vi "GenerateCode.vi"(1 "Terms":T1[](array[typedef]), 3 "Diagram":refnum<vi>, 5 "XRef":refnum<vi>, 6 "State In":T4={"Input Type"=variant(dbl 0.0), "Width"=0, "Typedef Name"="", "Value Type"=variant, "Selection"=0, "Options"=[], "Selections"=[], "Display Selections"=[], "Element Names"=[], "Typedef Name Width"=0, "Display Selection Width"=[], "Code Generated"=FALSE, "Is DVR"=FALSE, "Write Lock"=FALSE}) -> (0 "Generated Code?":bool, 2 "State Out":T4={"Input Type"=variant(dbl 0.0), "Width"=0, "Typedef Name"="", "Value Type"=variant, "Selection"=0, "Options"=[], "Selections"=[], "Display Selections"=[], "Element Names"=[], "Typedef Name Width"=0, "Display Selection Width"=[], "Code Generated"=FALSE, "Is DVR"=FALSE, "Write Lock"=FALSE}, 4 "Reply":string[](array[string]))   [LabVIEW 2015, in "Read-Write-Signals.xnode"]
doc: "This ability VI is called when it is time to define the execution behavior of your XNode via LabVIEW's scripting API. This VI is only called when you have previously informed LabVIEW that you need to script through a GenerateCode reply. Diagram is a reference to a diagram of a temporary VI. This diagram contains exactly one front panel terminal for each terminal of your XNode. Terms is an array of pairs of Term IDs and terminal references. LabVIEW will copy code scripted into this diagram into your XNode and connect everything to the correct terminals. The front panel terminals that are on this diagram are special in that they can only be on the top level diagram.\n \n Generate Code? is used to tell LabVIEW whether or not you want to copy the scripted diagram over. If there is an error and you wish not to commit the changes, then the old XNode behavior will be left unchanged. If you set Generate Code? to false, then this VI will be called again next time type propagation is run. Otherwise, it will not be called until you indicate that it should be through the reply on another ability VI.\n \n Because the diagram you are scripting into is separate from the VI containing the XNode instance, type propagation and the data manager will run on the temporary VI after each scripting call.\n \n You should not use the Copy scripting method to move code into the temporary VI. This will adversely affect the user's clipboard. You should use the Move scripting method instead.\n\nDefault behavior: None.\n\nThis ability does not provide UI and OS messages are not handled.\n\nSee also: ModifyCode"
uses:
  Read-Write-Signals.xnode
  State.ctl
  Read-Write-Signals Item.ctl
  Read-Write-Signals Sub Item.ctl
  Read-Write-Signals Sub Item Type.ctl
  Read-Write-Signals Selection.ctl
  Read-Write-Signals Display Selection.ctl
  <vilib>/XNodeSupport/XNodeTermIDPair.ctl
  <vilib>/XNodeSupport/XNodeTermRef.ctl
  <vilib>/XNodeSupport/XNodeString.ctl
  <vilib>/Erdos Miller/LV-Scripting/LV-Scripting.lvlib
  <vilib>/Utility/Data Type/NI_Data Type.lvlib
  <vilib>/XNodeSupport/NI_XNodeSupport.lvlib
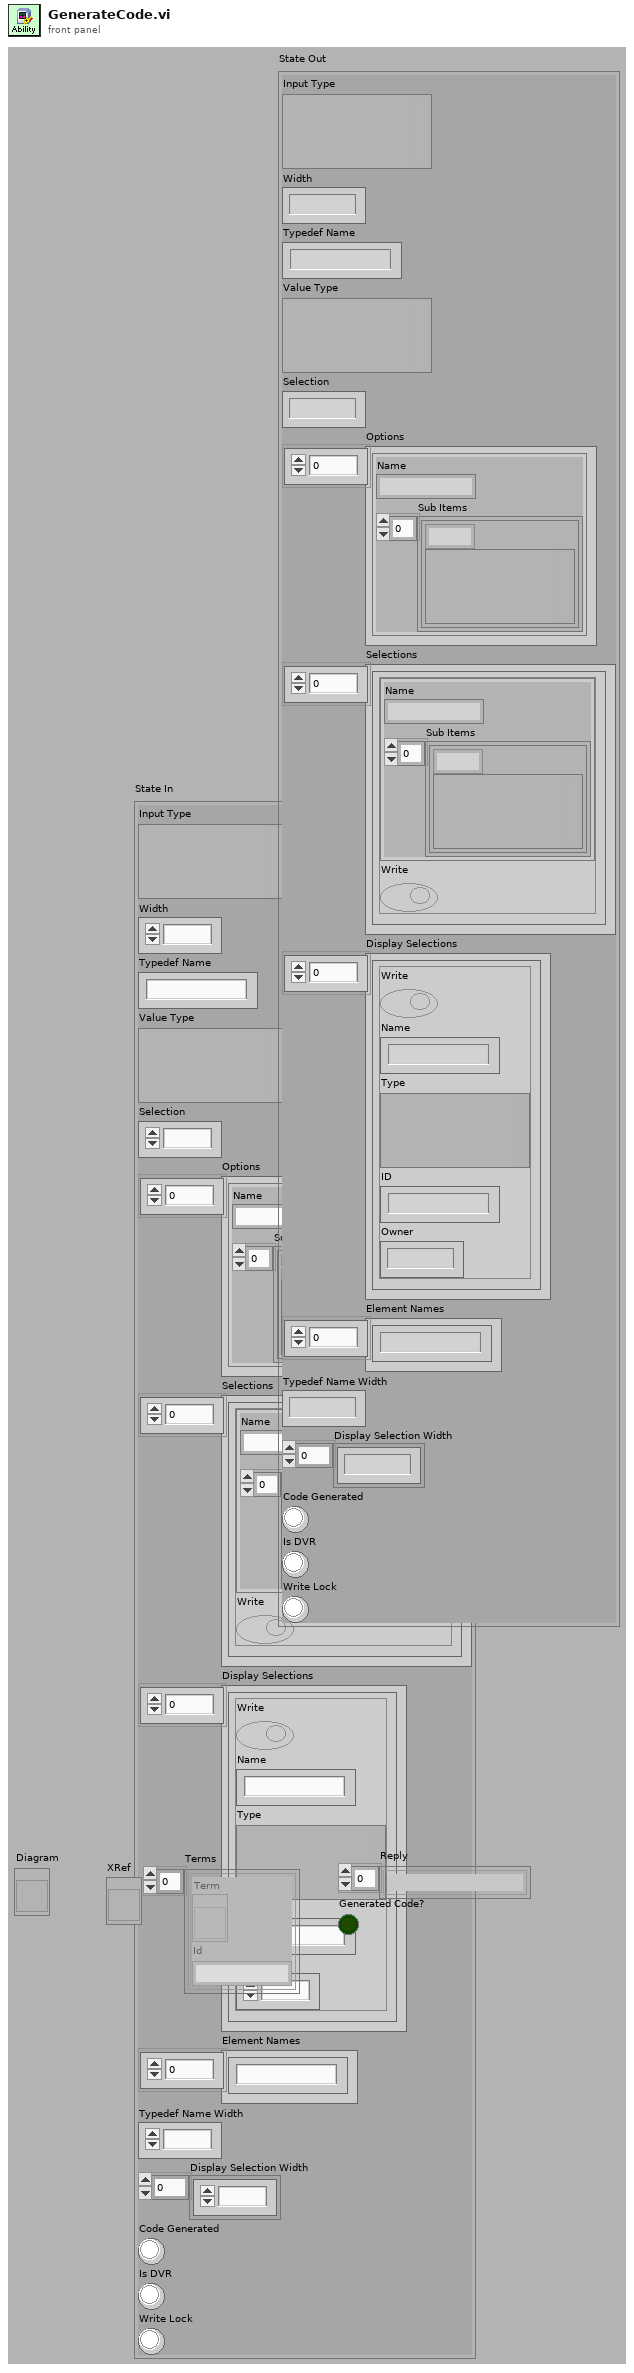
[diagram p1: front panel]
types:
  T1 = typedef "NI_XNodeSupport.lvlib/XNodeTermIDPair.ctl" = cluster{"Term":T2, "Id":T3}
  T2 = typedef "NI_XNodeSupport.lvlib/XNodeTermRef.ctl" = refnum<vi>
  T3 = typedef "NI_XNodeSupport.lvlib/XNodeString.ctl" = string
  T4 = typedef "Read-Write-Signals.xnode/State.ctl" = cluster{"Input Type":variant, "Width":i32, "Typedef Name":string, "Value Type":variant, "Selection":i32, "Options":T5[], "Selections":T8[], "Display Selections":T9[], "Element Names":string[], "Typedef Name Width":i32, "Display Selection Width":i32[], "Code Generated":bool, "Is DVR":bool, "Write Lock":bool}
  T5 = typedef "Read-Write-Signals Item.ctl" = cluster{"Name":string, "Sub Items":T6[]}
  T6 = typedef "Read-Write-Signals Sub Item.ctl" = cluster{"Type":T7, "Value":variant}
  T7 = typedef "Read-Write-Signals Sub Item Type.ctl" = enum8{"Cluster Element", "Array Element", "Subarray"}
  T8 = typedef "Read-Write-Signals Selection.ctl" = cluster{"Item":T5, "Write":bool}
  T9 = typedef "Read-Write-Signals Display Selection.ctl" = cluster{"Write":bool, "Name":string, "Type":variant, "ID":string, "Owner":i32}
  T10 = typedef "NI_Data Type.lvlib/Data Type.ctl" = enum8{"Invalid Type", "Void", "I8", "I16", "I32", "I64", "U8", "U16", "U32", "U64", "Single Float", "Double Float", "Extended Float", "Single Complex", "Double Complex", "Extended Complex", "Enum U8", "Enum U16", "Enum U32", "Enum U64", "Single Float With Unit", "Double Float With Unit", "Extended Float With Unit", "Single Complex with Unit", "Double Complex with Unit", "Extended Complex with Unit", "Boolean", "String", "Path", "Picture", "Tag", "Array", "Cluster", "Variant", "LV Variant", "Waveform", "Timestamp", "Digital Waveform", "Digital Data", "ExpressData", "Refnum", "External Data", "VI", "Poly VI", "LabVIEW Class Instance", "Fixed Point"}
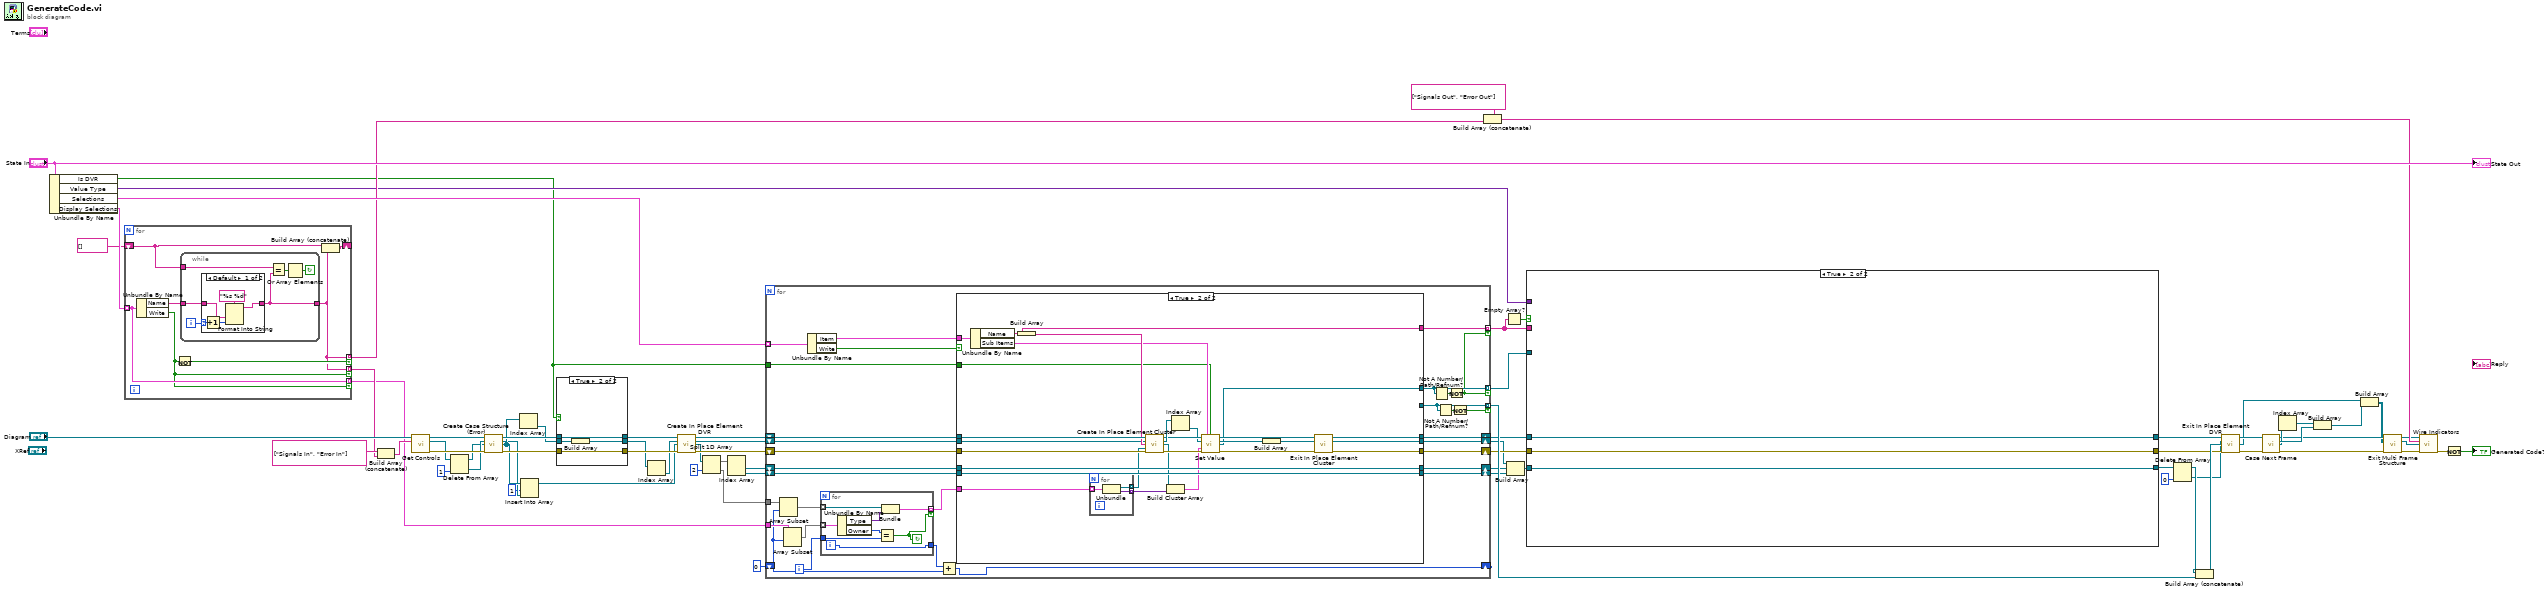
[diagram p0: block diagram]
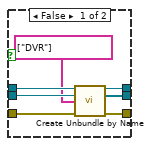
[diagram p2: hidden frame]
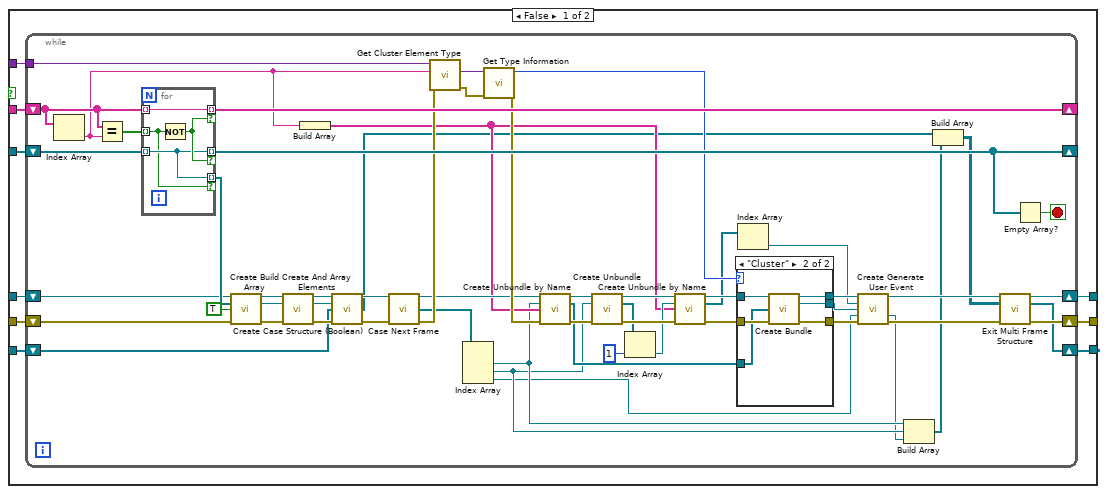
[diagram p3: hidden frame]
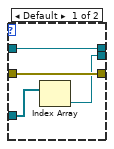
[diagram p4: hidden frame]
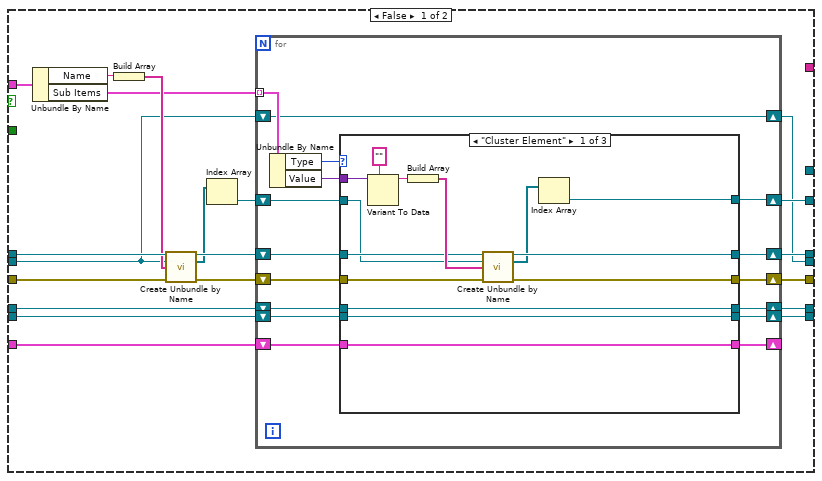
[diagram p5: hidden frame]
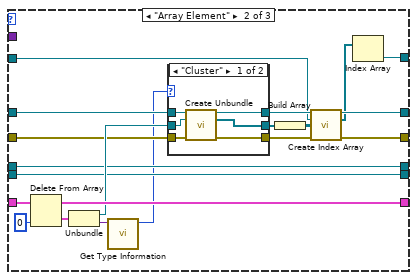
[diagram p6: hidden frame]
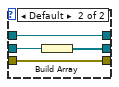
[diagram p7: hidden frame]
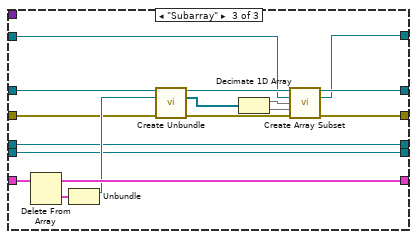
[diagram p8: hidden frame]
diagram:
  n1 = Unbundle By Name("State In") -> ("Is DVR"=w25:bool, "Value Type"=w41:variant, "Selections"=w63:T8[], "Display Selections"=w54:T9[])
  n2 = for {
    tunnel: w54 -> [w75] mode=indexing
    tunnel: [w76] -> w50 mode=indexing if=w80
    tunnel: [w76] -> w70 mode=indexing if=w74
    tunnel: [w75] -> w27 mode=indexing if=w74
    shift-right: [w79] -> _
    shift-left: string[] [] -> [w78]
    n3 = Unbundle By Name(w75) -> ("Name"=w77:string, "Write"=w74:bool)
    n4 = Not(x=w74) -> (.not. x?=w80:bool)
    n5 = while {
      tunnel: w77 -> [w84]
      tunnel: w78 -> [w86]
      tunnel: [w81] -> w76
      i -> [w85]
      stop <- w82 continue-if-true
      n6 = case shown="Default" w85 {
        selector: w85 -> [w90 _]
        tunnel: w84 -> [w89 w92]
        tunnel: [w88 w92] -> w81
        frame Default {
          n7 = Increment(x=w90) -> (x+1=w87:i32)
          n8 = Format Into String(format string="%s %d", w89, w87) -> (resulting string=w88:string)  [unwired: 2 in, 1 out]
        }
        frame 0 {
        }
      }
      n9 = Equal?(x=w86, y=w81) -> (x = y?=w83:bool[])
      n10 = Or Array Elements(Boolean array=w83) -> (logical OR=w82:bool)
    }
    n11 = Build Array (concatenate)(w78, w76) -> (w79:string[])
  }
  n12 = Build Array (concatenate)(string[] ["Signals In", "Error In"] ("Control Names"), w70) -> (w69:string[])
  n13 = call <vilib>:"Get Controls.vi"("Diagram in"="Diagram", "Control Names"=w69) -> ("Diagram out"=w23:refnum<vi>, "Control Terminals"=w18:refnum<vi>[], "error out"=w68:errorcluster)  [unwired: 11 in]
  n14 = Delete From Array(array=w18, index=1) -> (deleted portion=w21:refnum<vi>, array with subset deleted=w20:refnum<vi>[])  [unwired: 1 in]
  n15 = call <vilib>:"Create Case Structure (Error).vi"("Diagram in"=w23, "Selector"=w21, "Inputs"=w20, "error in (no error)"=w68) -> ("Selected Diagram"=w22:refnum<vi>, "Selector"=w3:refnum<vi>, "Inputs"=w4:refnum<vi>[], "error out"=w24:errorcluster)  [unwired: 8 in]
  n16 = Index Array(array=w4) -> (element=w19:refnum<vi>)  [unwired: 1 in]
  n17 = Insert Into Array(array=w4, index=1, new element=w3) -> (w1:refnum<vi>[])
  n18 = case shown="True" w25 {
    tunnel: w22 -> [w99 w103]
    tunnel: w24 -> [w98 w102]
    tunnel: w19 -> [w97 w101]
    tunnel: [w95 w103] -> w67
    tunnel: [w94 w102] -> w66
    tunnel: [w93 w100] -> w65
    frame False {
      n19 = call <vilib>:"Create Unbundle by Name.vi"("Diagram in"=w99, "input cluster"=w97, "Element Names"=string[] ["DVR"], "error in (no error)"=w98) -> ("Diagram out"=w95:refnum<vi>, "Outputs"=w93:refnum<vi>[], "error out"=w94:errorcluster)  [unwired: 9 in]
    }
    frame True {
      n20 = Build Array(w101) -> (w100:refnum<vi>[])
    }
  }
  n21 = Index Array(array=w65) -> (element=w64:refnum<vi>)  [unwired: 1 in]
  n22 = call <vilib>:"Create In Place Element DVR.vi"("Diagram in"=w67, "DVR"=w64, "Inputs"=w1, "error in (no error)"=w66) -> ("Diagram out"=w62:refnum<vi>, "Data Value"=w60:refnum<vi>, "Inputs"=w56:refnum<vi>[], "error out"=w61:errorcluster)  [unwired: 7 in, 1 out]
  n23 = Split 1D Array(array=w56, index=2) -> (first subarray=w55:refnum<vi>[], second subarray=w28:refnum<vi>[])
  n24 = Index Array(array=w55) -> (element #1=w58:refnum<vi>, element #2=w59:refnum<vi>)  [unwired: 2 in]
  n25 = for {
    tunnel: w63 -> [w131] mode=indexing
    shift-right: [w125] -> w42
    shift-left: w62 -> [w130]
    shift-right: [w124] -> w43
    shift-left: w61 -> [w129]
    shift-right: [w122] -> w39
    shift-left: w59 -> [w126]
    shift-right: [w123] -> w40
    shift-left: w58 -> [w127]
    tunnel: [w119] -> w53 mode=indexing if=w120
    shift-right: [w118] -> w38
    shift-left: w60 -> [w128]
    tunnel: [w116] -> w44 mode=indexing if=w114
    tunnel: [w115] -> w46 mode=indexing if=w114
    tunnel: w28 -> [w109]
    tunnel: w27 -> [w111]
    shift-right: [w107] -> _
    shift-left: 0 -> [w105]
    tunnel: w25 -> [w104]
    i -> [w113]
    n26 = Array Subset(array=w109, index=w105) -> (w108:refnum<vi>[])  [unwired: 1 in]
    n27 = Array Subset(array=w111, index=w105) -> (w110:T9[])  [unwired: 1 in]
    n28 = Unbundle By Name(w131) -> ("Item"=w132:T5, "Write"=w133:bool)
    n29 = for {
      tunnel: w108 -> [w137] mode=indexing
      tunnel: w110 -> [w141] mode=indexing
      tunnel: w113 -> [w139]
      tunnel: [w136] -> w112 mode=indexing if=w135
      tunnel: [w134] -> w106
      i -> [w134]
      stop <- w135 continue-if-true
      n30 = Unbundle By Name(w141) -> ("Type"=w138:variant, "Owner"=w140:i32)
      n31 = Equal?(x=w140, y=w139) -> (x = y?=w135:bool)
      n32 = Bundle(w137, "Type"=w138) -> (w136:cluster{refnum<vi>, "Type":variant})  [unwired: 1 in]
    }
    n33 = Add(x=w106, y=w105) -> (x+y=w107:i32)
    n34 = case shown="True" w133 {
      tunnel: w132 -> [w161 w265]
      tunnel: w130 -> [w160 w263]
      tunnel: w129 -> [w157 w261]
      tunnel: w128 -> [w143 w258]
      tunnel: w112 -> [w151 w245]
      tunnel: w127 -> [w150 w247]
      tunnel: w126 -> [w149 w248]
      tunnel: [w148 w256] -> w125
      tunnel: [w147 w257] -> w124
      tunnel: [w146 w247] -> w123
      tunnel: [w145 w248] -> w122
      tunnel: [w144 _] -> w119
      tunnel: [w142 w255] -> w118
      tunnel: [_ w241] -> w116
      tunnel: [_ w240] -> w115
      tunnel: w104 -> [_ w239]
      frame False {
        n35 = Unbundle By Name(w161) -> ("Name"=w159:string, "Sub Items"=w156:T6[])
        n36 = Build Array(w159) -> (w158:string[])
        n37 = call <vilib>:"Create Unbundle by Name.vi"("Diagram in"=w160, "input cluster"=w143, "Element Names"=w158, "error in (no error)"=w157) -> ("Diagram out"=w155:refnum<vi>, "Outputs"=w153:refnum<vi>[], "error out"=w154:errorcluster)  [unwired: 9 in]
        n38 = Index Array(array=w153) -> (element=w152:refnum<vi>)  [unwired: 1 in]
        n39 = for {
          tunnel: w156 -> [w177] mode=indexing
          shift-right: [w167] -> _
          shift-left: w151 -> [w174]
          shift-right: [w166] -> w148
          shift-left: w155 -> [w173]
          shift-right: [w165] -> w147
          shift-left: w154 -> [w172]
          shift-right: [w169] -> w146
          shift-left: w150 -> [w170]
          shift-right: [w168] -> w145
          shift-left: w149 -> [w171]
          shift-right: [w163] -> w144
          shift-left: w152 -> [w164]
          shift-right: [w162] -> w142
          shift-left: w143 -> [w162]
          n40 = Unbundle By Name(w177) -> ("Type"=w176:T7, "Value"=w175:variant)
          n41 = case shown="\"Cluster Element\"" w176 {
            tunnel: w175 -> [w189 _ _]
            tunnel: w174 -> [w178 w211 w238]
            tunnel: w173 -> [w185 w207 w234]
            tunnel: w172 -> [w184 w206 w233]
            tunnel: w171 -> [w190 w196 w232]
            tunnel: w170 -> [w191 w195 w231]
            tunnel: [w191 w195 w231] -> w169
            tunnel: [w190 w196 w232] -> w168
            tunnel: [w178 w210 w237] -> w167
            tunnel: [w183 w204 w228] -> w166
            tunnel: [w182 w203 w229] -> w165
            tunnel: w164 -> [w181 w199 w225]
            tunnel: [w179 w197 w227] -> w163
            frame "Cluster Element" {
              n42 = Variant To Data(type="", Variant=w189) -> (data=w187:string)  [unwired: 1 in, 1 out]
              n43 = Build Array(w187) -> (w186:string[])
              n44 = call <vilib>:"Create Unbundle by Name.vi"("Diagram in"=w185, "input cluster"=w181, "Element Names"=w186, "error in (no error)"=w184) -> ("Diagram out"=w183:refnum<vi>, "Outputs"=w180:refnum<vi>[], "error out"=w182:errorcluster)  [unwired: 9 in]
              n45 = Index Array(array=w180) -> (element=w179:refnum<vi>)  [unwired: 1 in]
            }
            frame "Array Element" {
              n46 = Delete From Array(array=w211, index=0) -> (deleted portion=w209:cluster{refnum<vi>, "Type":variant}, array with subset deleted=w210:cluster{refnum<vi>, "Type":variant}[])  [unwired: 1 in]
              n47 = Unbundle(w209) -> (w208:refnum<vi>, "Type"=w194:variant)
              n48 = call <vilib>:"Get Type Information.vi"("Variant"=w194) -> ("Type"=w193:T10)  [unwired: 6 in, 4 out]
              n49 = case shown="\"Cluster\"" w193 {
                tunnel: w208 -> [w215 w221]
                tunnel: w207 -> [w217 w219]
                tunnel: w206 -> [w216 w220]
                tunnel: [w213 w220] -> w202
                tunnel: [w214 w219] -> w201
                tunnel: [w212 w218] -> w200
                frame "Cluster" {
                  n50 = call <vilib>:"Create Unbundle.vi"("Diagram in"=w217, "input cluster"=w215, "error in (no error)"=w216) -> ("Diagram out"=w214:refnum<vi>, "Outputs"=w212:refnum<vi>[], "error out"=w213:errorcluster)  [unwired: 10 in]
                }
                frame Default {
                  n51 = Build Array(w221) -> (w218:refnum<vi>[])
                }
              }
              n52 = Build Array(w200) -> (w205:refnum<vi>[][])
              n53 = call <vilib>:"Create Index Array.vi"("Diagram in"=w201, "array"=w199, "Indices"=w205, "error in (no error)"=w202) -> ("Diagram out"=w204:refnum<vi>, "Outputs"=w198:refnum<vi>[], "error out"=w203:errorcluster)  [unwired: 9 in]
              n54 = Index Array(array=w198) -> (element=w197:refnum<vi>)  [unwired: 1 in]
            }
            frame "Subarray" {
              n55 = Delete From Array(array=w238) -> (deleted portion=w236:cluster{refnum<vi>, "Type":variant}, array with subset deleted=w237:cluster{refnum<vi>, "Type":variant}[])  [unwired: 2 in]
              n56 = Unbundle(w236) -> (w235:refnum<vi>)  [unwired: 1 out]
              n57 = call <vilib>:"Create Unbundle.vi"("Diagram in"=w234, "input cluster"=w235, "error in (no error)"=w233) -> ("Diagram out"=w226:refnum<vi>, "Outputs"=w224:refnum<vi>[], "error out"=w230:errorcluster)  [unwired: 10 in]
              n58 = Decimate 1D Array(w224) -> (w223:refnum<vi>[], w222:refnum<vi>[])
              n59 = call <vilib>:"Create Array Subset.vi"("Diagram in"=w226, "array"=w225, "Indices"=w223, "Lengths"=w222, "error in (no error)"=w230) -> ("Diagram out"=w228:refnum<vi>, "subarray"=w227:refnum<vi>, "error out"=w229:errorcluster)  [unwired: 8 in]
            }
          }
        }
      }
      frame True {
        n60 = Unbundle By Name(w265) -> ("Name"=w240:string, "Sub Items"=w254:T6[])
        n61 = Build Array(w240) -> (w259:string[])
        n62 = for {
          tunnel: w245 -> [w268] mode=indexing
          tunnel: [w267] -> w244 mode=indexing
          tunnel: [w266] -> w246 mode=indexing
          n63 = Unbundle(w268) -> (w267:refnum<vi>, "Type"=w266:variant)
        }
        n64 = call <vilib>:"Create In Place Element Cluster.vi"("Diagram in"=w263, "Cluster"=w258, "Element Names"=w259, "Inputs"=w244, "error in (no error)"=w261) -> ("Diagram out"=w253:refnum<vi>, "Elements"=w260:refnum<vi>[], "Inputs"=w243:refnum<vi>[], "error out"=w262:errorcluster)  [unwired: 7 in]
        n65 = Build Cluster Array(w243, w246) -> (w242:cluster{refnum<vi>, "Type":variant}[])
        n66 = Index Array(array=w260) -> (element=w252:refnum<vi>)  [unwired: 1 in]
        n67 = call "Set Value.vi"("Diagram in"=w253, "Sub Items"=w254, "Is DVR"=w239, "Value in"=w252, "Input Terms in"=w242, "error in (no error)"=w262) -> ("Diagram out"=w249:refnum<vi>, "Value out"=w251:refnum<vi>, "Equal"=w241:refnum<vi>, "error out"=w264:errorcluster)  [unwired: 5 in, 1 out]
        n68 = Build Array(w251) -> (w250:refnum<vi>[])
        n69 = call <vilib>:"Exit In Place Element Cluster.vi"("Diagram in"=w249, "Elements"=w250, "error in (no error)"=w264) -> ("Diagram out"=w256:refnum<vi>, "Cluster"=w255:refnum<vi>, "error out"=w257:errorcluster)  [unwired: 9 in, 1 out]
      }
    }
    n70 = Not A Number/Path/Refnum?(number/path/refnum=w116) -> (NaN/Path/Refnum?=w117:bool)
    n71 = Not A Number/Path/Refnum?(number/path/refnum=w119) -> (NaN/Path/Refnum?=w121:bool)
    n72 = Not(x=w117) -> (.not. x?=w114:bool)
    n73 = Not(x=w121) -> (.not. x?=w120:bool)
  }
  n74 = Build Array (concatenate)(string[] ["Signals Out", "Error Out"] ("Control Names"), w50) -> (w49:string[])
  n75 = Empty Array?(array=w46) -> (empty?=w45:bool)
  n76 = Build Array(w38, w40, w39) -> (w37:refnum<vi>[])
  n77 = case shown="True" w45 {
    tunnel: w46 -> [w277 _]
    tunnel: w44 -> [w276 _]
    tunnel: w43 -> [w275 w349]
    tunnel: w42 -> [w274 w348]
    tunnel: w37 -> [w273 w350]
    tunnel: w41 -> [w272 _]
    tunnel: [w271 w350] -> w34
    tunnel: [w270 w348] -> w36
    tunnel: [w269 w349] -> w35
    frame False {
      n78 = while {
        shift-right: [w331] -> _
        shift-left: w277 -> [w332]
        shift-right: [w328] -> _
        shift-left: w276 -> [w330]
        shift-right: [w289] -> w269
        shift-left: w275 -> [w325]
        shift-right: [w279] -> w270
        shift-left: w274 -> [w318]
        shift-right: [w280] -> w271
        shift-left: w273 -> [w281]
        tunnel: w272 -> [w317]
        stop <- w329 stop-if-true
        n79 = Index Array(array=w332) -> (element=w306:string)  [unwired: 1 in]
        n80 = Equal?(x=w332, y=w306) -> (x = y?=w333:bool[])
        n81 = for {
          tunnel: w333 -> [w344] mode=indexing
          tunnel: w332 -> [w347] mode=indexing
          tunnel: [w347] -> w331 mode=indexing if=w346
          tunnel: w330 -> [w345] mode=indexing
          tunnel: [w345] -> w328 mode=indexing if=w346
          tunnel: [w345] -> w327 mode=indexing if=w344
          n82 = Not(x=w344) -> (.not. x?=w346:bool)
        }
        n83 = call <vilib>:"Create Build Array.vi"("Diagram in"=w318, "Inputs"=w327, "Concatenate Inputs"=TRUE, "error in (no error)"=w325) -> ("Diagram out"=w322:refnum<vi>, "appended array"=w321:refnum<vi>, "error out"=w324:errorcluster)  [unwired: 9 in]
        n84 = call <vilib>:"Create And Array Elements.vi"("Diagram in"=w322, "Boolean array"=w321, "error in (no error)"=w324) -> ("Diagram out"=w320:refnum<vi>, "logical AND"=w319:refnum<vi>, "error out"=w323:errorcluster)  [unwired: 10 in]
        n85 = Build Array(w306) -> (w297:string[])
        n86 = call <vilib>:"Create Case Structure (Boolean).vi"("Diagram in"=w320, "Selector"=w319, "Inputs"=w281, "error in (no error)"=w323) -> ("Selected Diagram"=w309:refnum<vi>, "Inputs"=w284:refnum<vi>[], "error out"=w316:errorcluster)  [unwired: 8 in, 1 out]
        n87 = call <vilib>:"Case Next Frame.vi"("Diagram in"=w309, "error in (no error)"=w316) -> ("Selected Diagram"=w308:refnum<vi>, "Inputs"=w307:refnum<vi>[], "error out"=w310:errorcluster)  [unwired: 10 in, 1 out]
        n88 = call <vilib>:"Get Cluster Element Type.vi"("error in (no error)"=w310, "Element Name"=w306, "Cluster in"=w317) -> ("error out"=w314:errorcluster, "Type"=w315:variant)  [unwired: 6 in, 1 out]
        n89 = Index Array(array=w307) -> (element #1=w287:refnum<vi>, element #2=w286:refnum<vi>, element #3=w285:refnum<vi>)  [unwired: 3 in]
        n90 = call <vilib>:"Get Type Information.vi"("error in (no error)"=w314, "Variant"=w315) -> ("error out"=w312:errorcluster, "Type"=w313:T10)  [unwired: 5 in, 3 out]
        n91 = call <vilib>:"Create Unbundle by Name.vi"("Diagram in"=w308, "input cluster"=w287, "Element Names"=w297, "error in (no error)"=w312) -> ("Diagram out"=w304:refnum<vi>, "Outputs"=w292:refnum<vi>[], "error out"=w305:errorcluster)  [unwired: 9 in]
        n92 = call <vilib>:"Create Unbundle.vi"("Diagram in"=w304, "input cluster"=w286, "error in (no error)"=w305) -> ("Diagram out"=w301:refnum<vi>, "Outputs"=w300:refnum<vi>[], "error out"=w303:errorcluster)  [unwired: 10 in]
        n93 = Index Array(array=w300, index=1) -> (element=w298:refnum<vi>)
        n94 = call <vilib>:"Create Unbundle by Name.vi"("Diagram in"=w301, "input cluster"=w298, "Element Names"=w297, "error in (no error)"=w303) -> ("Diagram out"=w296:refnum<vi>, "Outputs"=w291:refnum<vi>[], "error out"=w302:errorcluster)  [unwired: 9 in]
        n95 = case shown="\"Cluster\"" w313 {
          tunnel: w302 -> [w337 w343]
          tunnel: [w337 w342] -> w311
          tunnel: w296 -> [w336 w341]
          tunnel: [w336 w340] -> w294
          tunnel: [w335 w339] -> w293
          tunnel: w292 -> [w334 w338]
          frame Default {
            n96 = Index Array(array=w334) -> (element=w335:refnum<vi>)  [unwired: 1 in]
          }
          frame "Cluster" {
            n97 = call <vilib>:"Create Bundle.vi"("Diagram in"=w341, "Inputs"=w338, "error in (no error)"=w343) -> ("Diagram out"=w340:refnum<vi>, "output cluster"=w339:refnum<vi>, "error out"=w342:errorcluster)  [unwired: 10 in]
          }
        }
        n98 = Index Array(array=w291) -> (element=w290:refnum<vi>)  [unwired: 1 in]
        n99 = call <vilib>:"Create Generate User Event.vi"("Diagram in"=w294, "user event"=w290, "event data cluster"=w293, "error in"=w285, "error in (no error)"=w311) -> ("Diagram out"=w288:refnum<vi>, 10:"error out"=w278:refnum<vi>, 15:"error out"=w295:errorcluster)  [unwired: 7 in, 1 out]
        n100 = Build Array(w287, w286, w278) -> (w283:refnum<vi>[])
        n101 = Build Array(w284, w283) -> (w282:refnum<vi>[][])
        n102 = call <vilib>:"Exit Multi Frame Structure.vi"("Diagram in"=w288, "Outputs"=w282, "error in (no error)"=w295) -> ("Diagram out"=w279:refnum<vi>, "Outputs"=w280:refnum<vi>[], "error out"=w289:errorcluster)  [unwired: 10 in]
        n103 = Empty Array?(array=w328) -> (empty?=w329:bool)
      }
    }
    frame True {
    }
  }
  n104 = Delete From Array(array=w34, index=0) -> (deleted portion=w31:refnum<vi>, array with subset deleted=w33:refnum<vi>[])  [unwired: 1 in]
  n105 = Build Array (concatenate)(w33, w53) -> (w52:refnum<vi>[])
  n106 = call <vilib>:"Exit In Place Element DVR.vi"("Diagram in"=w36, "Data Value"=w31, "Outputs"=w52, "error in (no error)"=w35) -> ("Diagram out"=w16:refnum<vi>, "Outputs"=w13:refnum<vi>[], "error out"=w48:errorcluster)  [unwired: 7 in, 2 out]
  n107 = call <vilib>:"Case Next Frame.vi"("Diagram in"=w16, "error in (no error)"=w48) -> ("Selected Diagram"=w10:refnum<vi>, "Selector"=w15:refnum<vi>, "Inputs"=w14:refnum<vi>[], "error out"=w17:errorcluster)  [unwired: 10 in]
  n108 = Index Array(array=w14) -> (element=w5:refnum<vi>)  [unwired: 1 in]
  n109 = Build Array(w5, w15) -> (w12:refnum<vi>[])
  n110 = Build Array(w13, w12) -> (w8:refnum<vi>[][])
  n111 = call <vilib>:"Exit Multi Frame Structure.vi"("Diagram in"=w10, "Outputs"=w8, "error in (no error)"=w17) -> ("Diagram out"=w9:refnum<vi>, "Outputs"=w7:refnum<vi>[], "error out"=w11:errorcluster)  [unwired: 10 in]
  n112 = call <vilib>:"Wire Indicators.vi"("Diagram in"=w9, "Indicator Names"=w49, "Outputs"=w7, "error in (no error)"=w11) -> ("error out"=w29:errorcluster)  [unwired: 10 in, 1 out]
  n113 = Not(x=w29) -> (.not. x?=→"Generated Code?":bool)
  "State Out" <- "State In"
